vi "parse_KH_string.vi"() -> ()   [LabVIEW 2013]
panel:
  out "Measurement Type":string[](array[string])
  out "Gain":dbl[](array[numeric])
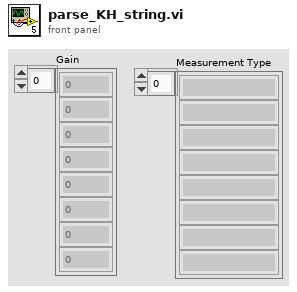
[diagram p1: front panel]
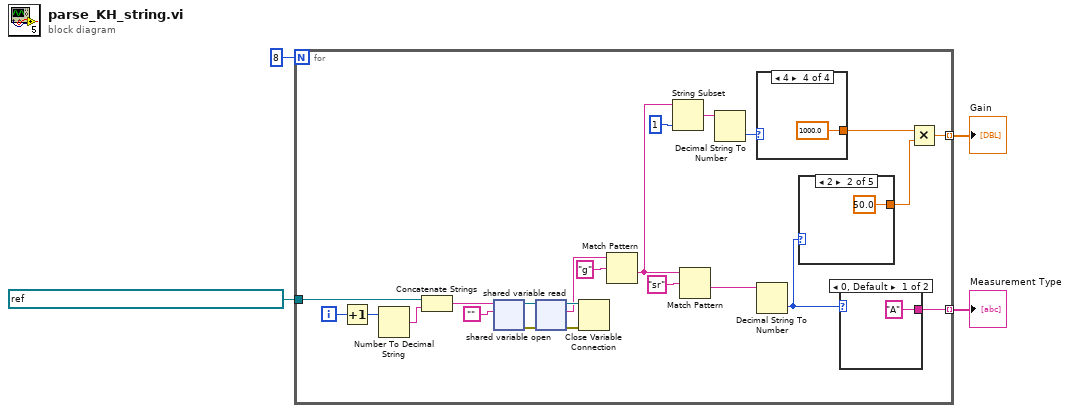
[diagram p0: block diagram]
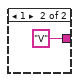
[diagram p2: hidden frame]
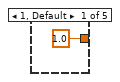
[diagram p3: hidden frame]
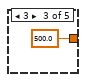
[diagram p4: hidden frame]
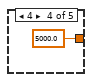
[diagram p5: hidden frame]
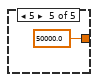
[diagram p6: hidden frame]
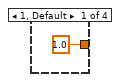
[diagram p7: hidden frame]
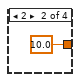
[diagram p8: hidden frame]
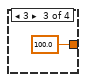
[diagram p9: hidden frame]
diagram:
  n1 = for {
    N: 8 -> [_]
    tunnel: refnum<k21> "ni.var.psp://housesoftheholy/MNK_18T/KH_ch" ("shared variable refnum in") -> [w26]
    tunnel: [w7] -> w3 mode=indexing
    tunnel: [w6] -> w2 mode=indexing
    i -> [w25]
    n2 = Increment(x=w25) -> (x+1=w24:i32)
    n3 = Number To Decimal String(number=w24) -> (decimal integer string=w23:string)  [unwired: 1 in]
    n4 = Concatenate Strings(w26, w23) -> (w22:string)
    n5 = shared-variable-open(w22, "") -> (w20:refnum<k21>, w5:errorcluster)  [unwired: 2 in]
    n6 = shared-variable-read(w20, w5) -> (w19:refnum<k21>, w27:errorcluster, w8:string)  [unwired: 1 out]
    n7 = Close Variable Connection(8:w27, 11:w19) -> ()  [unwired: 1 out]
    n8 = Match Pattern(string=w8, regular expression="g") -> (after substring=w11:string)  [unwired: 1 in, 3 out]
    n9 = String Subset(string=w11, length (rest)=1 ("length (rest)")) -> (substring=w13:string)  [unwired: 1 in]
    n10 = Match Pattern(string=w11, regular expression="sr") -> (after substring=w15:string)  [unwired: 1 in, 3 out]
    n11 = Decimal String To Number(string=w13) -> (number=w14:i32)  [unwired: 2 in, 1 out]
    n12 = case shown="4" w14 {
      tunnel: [1.0 10.0 100.0 1000.0] -> w16
      frame 1, Default {
      }
      frame 2 {
      }
      frame 3 {
      }
      frame 4 {
      }
    }
    n13 = Decimal String To Number(string=w15) -> (number=w18:i32)  [unwired: 2 in, 1 out]
    n14 = case shown="2" w18 {
      tunnel: [1.0 50.0 500.0 5000.0 50000.0] -> w17
      frame 1, Default {
      }
      frame 2 {
      }
      frame 3 {
      }
      frame 4 {
      }
      frame 5 {
      }
    }
    n15 = case shown="0, Default" w18 {
      tunnel: ["A" "V"] -> w6
      frame 0, Default {
      }
      frame 1 {
      }
    }
    n16 = Multiply(x=w16, y=w17) -> (x*y=w7:dbl)
  }
  "Gain" <- w3
  "Measurement Type" <- w2
